vi "SendPacket.vi"(6 "timeout (1000ms)":i32=1000, 8 "error in (no error)":errorcluster, 9 "Wait for ack? (T)":bool=TRUE, 10 "ControlPacket":refnum<class "ControlPacket.lvclass">, 11 "Client in":refnum<class "Client.lvclass">) -> (0 "error out":errorcluster, 2 "Response":refnum<class "ControlPacket.lvclass">[](array[class]), 3 "Client out":refnum<class "Client.lvclass">)   [LabVIEW 2013, in "MQTT Client.lvlib" / "Client.lvclass"]
uses:
  Client.lvclass
  <vilib>/LabVIEW Open Source Project/MQTT Control Packets/Control Packets/ControlPacket/ControlPacket.lvclass
  <vilib>/LabVIEW Open Source Project/MQTT Control Packets/Control Packets/ControlPacket/ControlPacket.lvclass/ControlPacket.ctl
  Session.Client/Session.Client.lvclass
  <vilib>/LabVIEW Open Source Project/MQTT Connection/MQTT_Base/Session/Session.lvclass
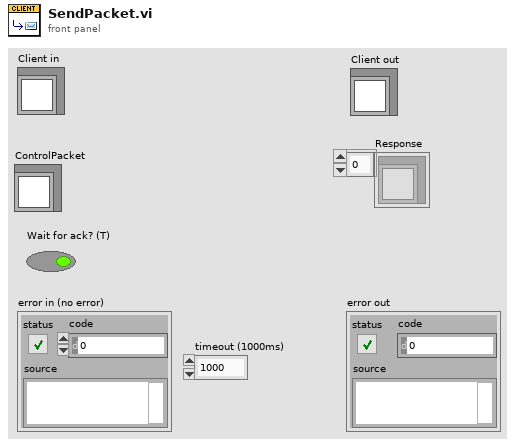
[diagram p1: front panel]
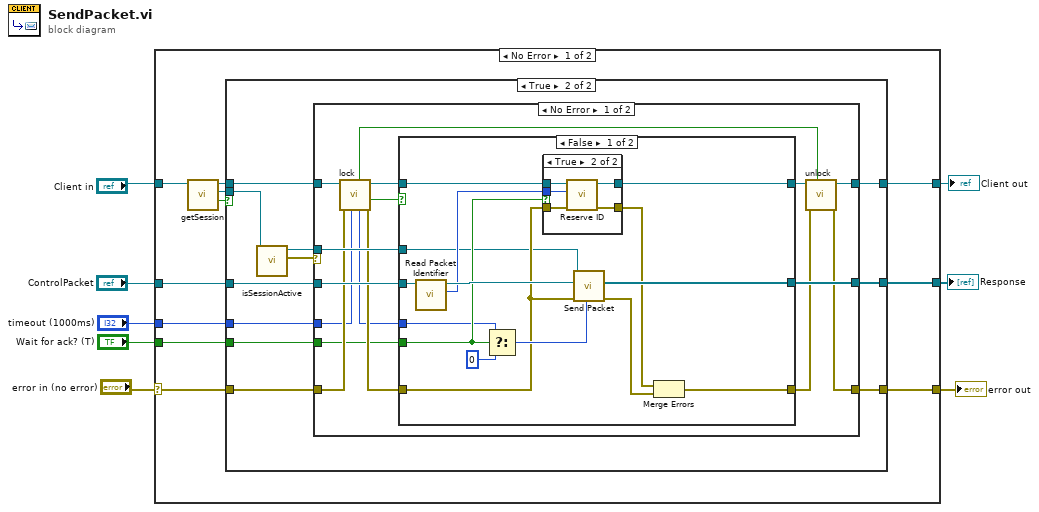
[diagram p0: block diagram]
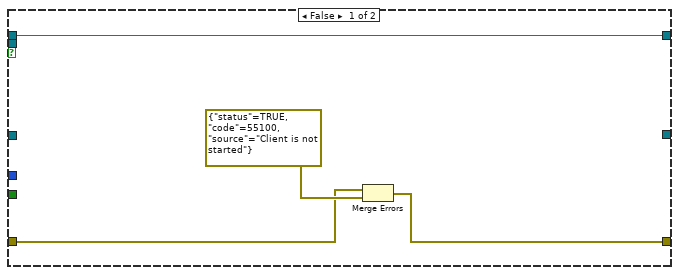
[diagram p2: hidden frame]
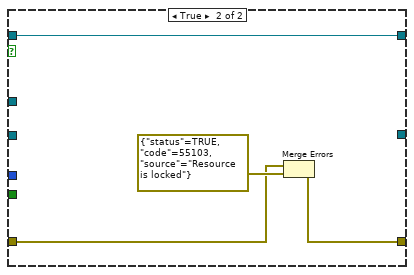
[diagram p4: hidden frame]
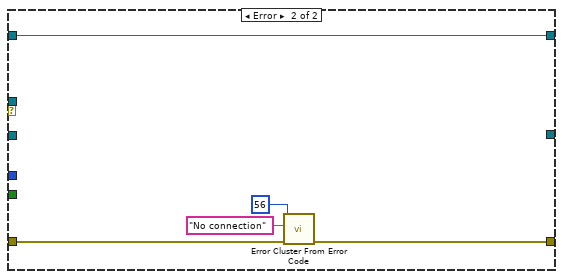
[diagram p5: hidden frame]
diagram:
  n1 = case shown="No Error" "error in (no error)" {
    selector: "error in (no error)" -> [w19 w83]
    tunnel: [w15 w83] -> w5
    tunnel: [w14 w82] -> w6
    tunnel: "Client in" -> [w12 w82]
    tunnel: "ControlPacket" -> [w17 _]
    tunnel: [w18 _] -> w3
    tunnel: "timeout (1000ms)" -> [w16 _]
    tunnel: "Wait for ack? (T)" -> [w9 _]
    frame No Error {
      n2 = call "getSession.vi"("Client in"=w12) -> ("valid?"=w10:bool, "Session"=w13:refnum<class "Session.Client.lvclass">, "Client out"=w11:refnum<class "Client.lvclass">)  [unwired: 8 in]
      n3 = case shown="True" w10 {
        tunnel: w19 -> [w21 w34]
        tunnel: [_ w33] -> w18
        tunnel: w17 -> [_ w32]
        tunnel: w16 -> [_ w31]
        tunnel: [w20 w30] -> w15
        tunnel: [w23 w28] -> w14
        tunnel: w13 -> [_ w24]
        tunnel: w11 -> [w23 w27]
        tunnel: w9 -> [_ w26]
        frame False {
          n4 = Merge Errors(w21, errorcluster {"status"=TRUE, "code"=55100, "source"="Client is not started"} ("error in")) -> (w20:errorcluster)
        }
        frame True {
          n5 = call <vilib>:"isSessionActive.vi"("Session in"=w24) -> ("error out"=w29:errorcluster, "Session out"=w25:refnum<class "Session.Client.lvclass">)  [unwired: 9 in]
          n6 = case shown="No Error" w29 {
            tunnel: w34 -> [w42 w78]
            tunnel: [w50 _] -> w33
            tunnel: w32 -> [w49 _]
            tunnel: w31 -> [w40 _]
            tunnel: [w44 w77] -> w30
            tunnel: w27 -> [w47 w81]
            tunnel: w25 -> [w48 _]
            tunnel: [w46 w81] -> w28
            tunnel: w26 -> [w37 _]
            frame No Error {
              n7 = call "lock.vi"("timeout (2000ms)"=w40, "error in (no error)"=w42, "Client in"=w47) -> ("error out"=w41:errorcluster, "timed out"=w38:bool, "Client out"=w36:refnum<class "Client.lvclass">, "remaining (ms)"=w39:i32, "locked"=w43:bool)  [unwired: 4 in]
              n8 = case shown="False" w38 {
                tunnel: [w65 _] -> w50
                tunnel: w49 -> [w64 _]
                tunnel: w48 -> [w53 _]
                tunnel: [w61 w74] -> w45
                tunnel: w41 -> [w55 w75]
                tunnel: w39 -> [w52 _]
                tunnel: w37 -> [w54 _]
                tunnel: w36 -> [w58 w73]
                tunnel: [w57 w73] -> w35
                frame False {
                  n9 = call <vilib>:"Read Packet Identifier.vi"("ControlPacket in"=w64) -> ("Packet Identifier"=w59:u16, "ControlPacket out"=w63:refnum<class "ControlPacket.lvclass">)  [unwired: 9 in]
                  n10 = Select(t=w52, s=w54, f=0) -> (s? t:f=w60:i32)
                  n11 = case shown="True" w54 {
                    tunnel: w59 -> [_ w72]
                    tunnel: w58 -> [w67 w71]
                    tunnel: [w67 w70] -> w57
                    tunnel: [w66 w69] -> w56
                    tunnel: w55 -> [w66 w68]
                    frame False {
                    }
                    frame True {
                      n12 = call "Reserve ID.vi"("error in (no error)"=w68, "Packet Identifier"=w72, "Client in"=w71) -> ("error out"=w69:errorcluster, "Client out"=w70:refnum<class "Client.lvclass">)  [unwired: 7 in]
                    }
                  }
                  n13 = call "Send Packet.vi"("timeout (0ms : no ack)"=w60, "error in (no error)"=w55, "Packet"=w63, "Session"=w53) -> ("error out"=w62:errorcluster, "Response"=w65:refnum<class "ControlPacket.lvclass">[])  [unwired: 4 in, 2 out]
                  n14 = Merge Errors(w56, w62) -> (w61:errorcluster)
                }
                frame True {
                  n15 = Merge Errors(w75, errorcluster {"status"=TRUE, "code"=55103, "source"="Resource is locked"} ("error in")) -> (w74:errorcluster)
                }
              }
              n16 = call "unlock.vi"("Unlock?"=w43, "error in (no error)"=w45, "Client in"=w35) -> ("error out"=w44:errorcluster, "Client out"=w46:refnum<class "Client.lvclass">)  [unwired: 7 in]
            }
            frame Error {
              n17 = call <vilib>:"Error Cluster From Error Code.vi"("error in (no error)"=w78, "error message (\"\")"="No connection" ("error message (\"\")"), "error code (0)"=56) -> ("error out"=w77:errorcluster)  [unwired: 6 in]
            }
          }
        }
      }
    }
    frame Error {
    }
  }
  "error out" <- w5
  "Client out" <- w6
  "Response" <- w3
